vi "startILC.vi"(8 "error in (no error)":errorcluster, 11 "ILC in":refnum<class "ILC.lvclass">) -> (0 "error out":errorcluster, 3 "ILC out":refnum<class "ILC.lvclass">)   [LabVIEW 2013]
uses:
  <userlib>/Common/ILC/ILC/ILC.lvclass
  <userlib>/Common/SerialProtocols/SerialCommunicator/SerialCommunicator.lvclass
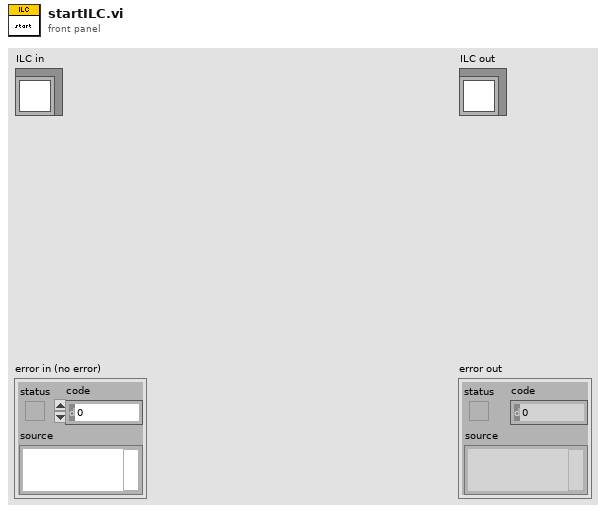
[diagram p1: front panel]
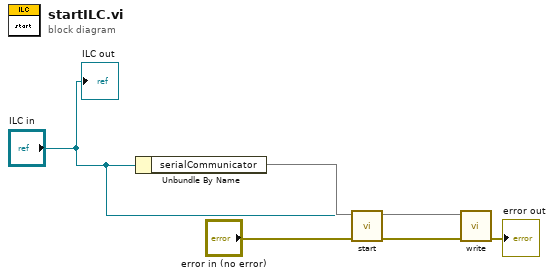
[diagram p0: block diagram]
diagram:
  n1 = Unbundle By Name("ILC in") -> ("serialCommunicator"=w5)
  n2 = call <userlib>:"start.vi"("error in (no error)"="error in (no error)", "ILC in"="ILC in") -> ("error out"=w2:errorcluster)  [unwired: 8 in, 1 out]
  n3 = call-dynamic "write.vi"("error in (no error)"=w2, "SerialCommunicator in"=w5) -> ("error out"=→"error out":errorcluster)  [unwired: 8 in, 1 out]
  "ILC out" <- "ILC in"
